vi "Is CSM Module - Structure.vi"(8 "error in (no error)":errorcluster, 11 "Structure":refnum<vi>) -> (0 "error out":errorcluster, 2 "Is CSM Module?":bool, 3 "CSM Basic Refs":T1)   [LabVIEW 2017, in "CSM-Helper Utility.lvlib"]
doc: "#### Is CSM Module - Structure.vi\n\nDetermine if it is a CSM module through Structure reference\n\n-- <b>Controls</b> --\n- <b>Structure</b>: Structure reference\n\n-- <b>Indicators</b> --\n- <b>Is CSM Module?</b>: True If it is a CSM module\n- <b>CSM Basic Refs</b>: If This is a CSM module, It will return the basic references"
uses:
  CSM-Helper Utility.lvlib
  CSM Basic Refs.ctl
  CSM Module Type.ctl
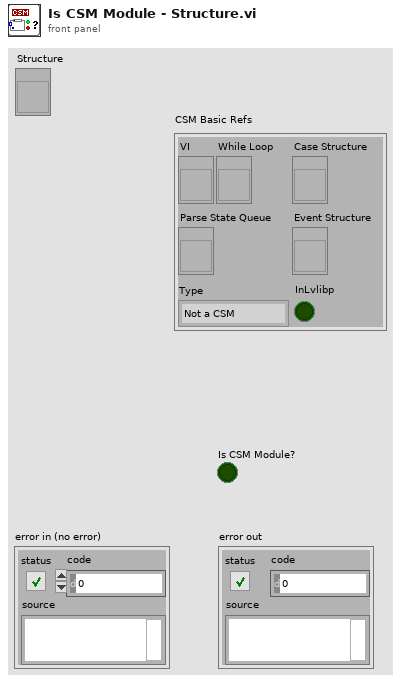
[diagram p1: front panel]
types:
  T1 = typedef "CSM-Helper Utility.lvlib/CSM Basic Refs.ctl" = cluster{"VI":refnum<vi>, "While Loop":refnum<vi>, "Case Structure":refnum<vi>, "Parse State Queue":refnum<vi>, "Event Structure":refnum<vi>, "Type":T2, "InLvlibp":bool}
  T2 = typedef "CSM-Helper Utility.lvlib/CSM Module Type.ctl" = enum16{"Not a CSM", "JKISM", "CSM"}
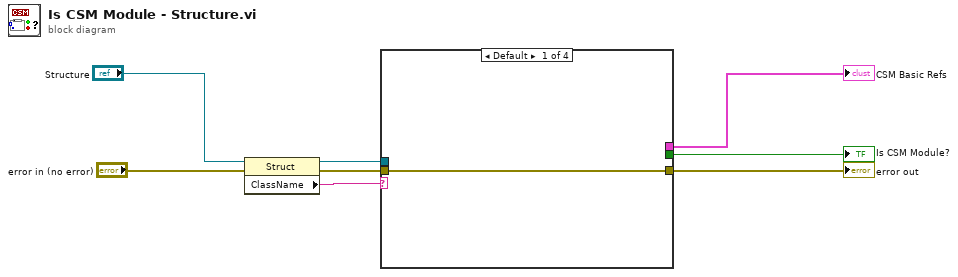
[diagram p0: block diagram]
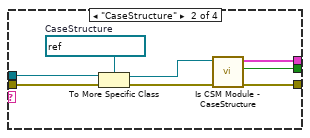
[diagram p2: hidden frame]
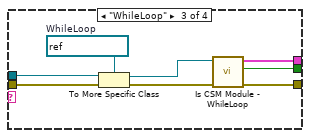
[diagram p3: hidden frame]
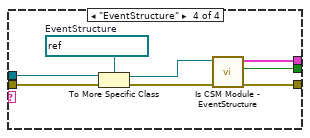
[diagram p4: hidden frame]
diagram:
  n1 = property class="Struct"(reference="Structure", error in="error in (no error)") -> (reference out=w4:refnum<vi>, error out=w6:errorcluster, "ClassName"=w1:string)
  n2 = case shown="Default" w1 {
    tunnel: w6 -> [w9 w17 w25 w33]
    tunnel: [w9 w16 w24 w32] -> w5
    tunnel: w4 -> [_ w12 w20 w28]
    tunnel: [_ w15 w23 w31] -> w3
    tunnel: [_ w14 w22 w30] -> w2
    frame Default {
    }
    frame "CaseStructure" {
      w11 = refnum<vi> refnum  # CaseStructure
      n3 = To More Specific Class(target class=w11, reference=w12, error in=w17) -> (specific class reference=w10:refnum<vi>, error out=w13:errorcluster)
      n4 = call "Is CSM Module - CaseStructure.vi"("error in (no error)"=w13, "CaseStructure"=w10) -> ("error out"=w16:errorcluster, "Is CSM Module?"=w14:bool, "CSM Basic Refs"=w15:T1)  [unwired: 7 in]
    }
    frame "WhileLoop" {
      w19 = refnum<vi> refnum  # WhileLoop
      n5 = To More Specific Class(target class=w19, reference=w20, error in=w25) -> (specific class reference=w18:refnum<vi>, error out=w21:errorcluster)
      n6 = call "Is CSM Module - WhileLoop.vi"("error in (no error)"=w21, "WhileLoop in"=w18) -> ("error out"=w24:errorcluster, "Is CSM Module?"=w22:bool, "CSM Basic Refs"=w23:T1)  [unwired: 6 in, 1 out]
    }
    frame "EventStructure" {
      w27 = refnum<vi> refnum  # EventStructure
      n7 = To More Specific Class(target class=w27, reference=w28, error in=w33) -> (specific class reference=w26:refnum<vi>, error out=w29:errorcluster)
      n8 = call "Is CSM Module - EventStructure.vi"("error in (no error)"=w29, "EventStructure"=w26) -> ("error out"=w32:errorcluster, "Is CSM Module?"=w30:bool, "CSM Basic Refs"=w31:T1)  [unwired: 7 in]
    }
  }
  "error out" <- w5
  "CSM Basic Refs" <- w3
  "Is CSM Module?" <- w2
